vi "Flatten.vi"(8 "error in":errorcluster, 9 "Data":T1) -> (0 "error out":errorcluster, 2 "Buffer":u8[](array[numeric]) format="%.0x")   [LabVIEW 2020, in "Service.lvlib"]
uses:
  Service.lvlib
  Data.ctl
  ServiceType/Enumeration.ctl
  <vilib>/IlluminatedG/IG Protoc/LV-Proto/Wire Encode Tag.vi
  ServiceType/Enum Value.vi
  <vilib>/IlluminatedG/IG Protoc/LV-Proto/Wire Encode Varint I32.vi
  ServiceType/ServiceType.lvlib
  <vilib>/IlluminatedG/IG Protoc/LV-Proto/LV-Proto.lvlib
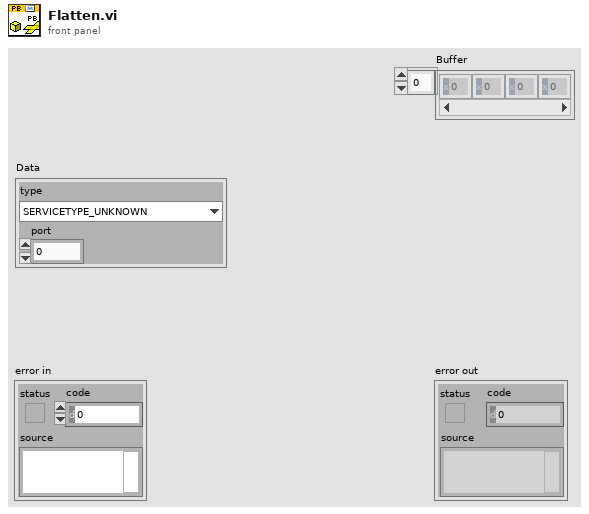
[diagram p1: front panel]
types:
  T1 = typedef "Service.lvlib/Data.ctl" = cluster{"type":T2, "port":i32}
  T2 = typedef "ServiceType.lvlib/Enumeration.ctl" = enum16{"SERVICETYPE_UNKNOWN", "SERVICETYPE_TCPSERVER", "SERVICETYPE_HTTPSERVER"}
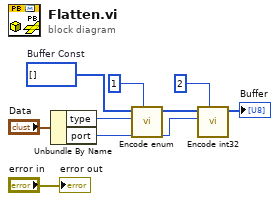
[diagram p0: block diagram]
diagram:
  w7 = u8[] []  # Buffer Const
  n1 = Unbundle By Name("Data") -> ("type"=w5:T2, "port"=w2:i32)
  n2 = call "Encode enum.vi"("Field Number"=1, "Enumeration"=w5, "Buffer in"=w7) -> ("Buffer"=w4:u8[])  [unwired: 8 in]
  n3 = call <vilib>:"Encode int32.vi"("Field Number"=2, "int32"=w2, "Buffer in"=w4) -> ("Buffer"=→"Buffer":u8[])  [unwired: 8 in]
  "error out" <- "error in"
